vi "Configure Measurement Trend (TIE).vi"(0 "VISA resource name":refnum<visa-resource-name>, 1 "Enable Measurement Trend (T:Enable)":bool, 2 "Direction (0: Rising)":i32(ring) items=["Rising", "Falling", "Both"], 3 "Units (0: Second)":i32(ring) items=["Second", "Unit Interval"], 5 "Source 1 (1: Channel 1)":i32(ring) items=["Channel 1", "Channel 2", "Channel 3", "Channel 4", "Function 1", "Function 2", "Function 3", "Function 4", "Memory 1", "Memory 2", "Memory 3", "Memory 4"], 9 "Measurement Function (0: Time Interval Error (Data))":i32(ring) items=["Time Interval Error (Data)", "Time Interval Error (Clock)"], 11 "error in (no error)":errorcluster) -> (4 "VISA resource name out":refnum<visa-resource-name>, 15 "error out":errorcluster)   [LabVIEW 2009, in "Agilent 8000 Series.lvlib"]
doc: "Configures either Time Interval Error measurement and enables the Measurement Trend Jitter analysis on it.\n\n<B>Note:</B>\nCalling this VI disables all previously enabled measurements and clears existing measurement results from display."
uses:
  Agilent 8000 Series.lvlib
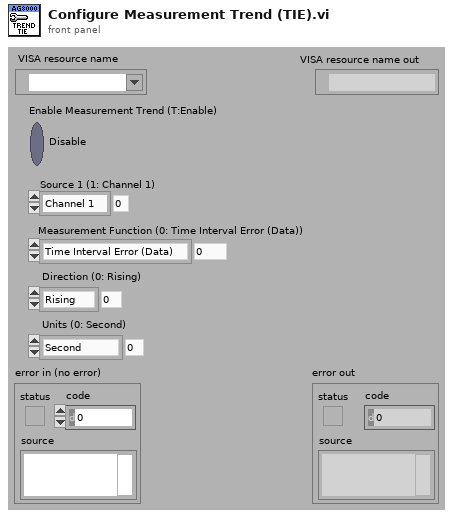
[diagram p1: front panel]
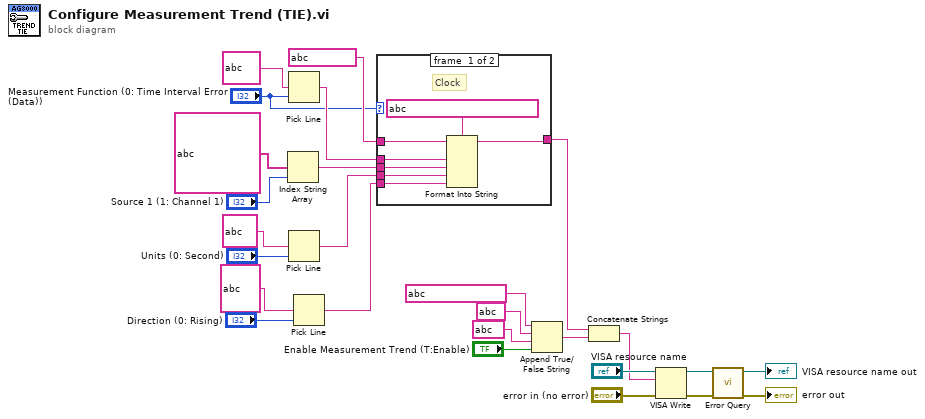
[diagram p0: block diagram]
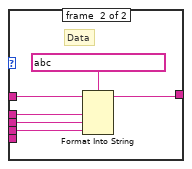
[diagram p2: hidden frame]
diagram:
  n1 = Index String Array(1:"Source 1 (1: Channel 1)", 2:string[] ?) -> (0:w15:string)  [unwired: 1 in]
  n2 = Pick Line(multi-line string=string ?, line index="Measurement Function (0: Time Interval Error (Data))") -> (output string=w18:string)  [unwired: 1 in]
  n3 = Pick Line(multi-line string=string ?, line index="Units (0: Second)") -> (output string=w9:string)  [unwired: 1 in]
  n4 = Pick Line(multi-line string=string ?, line index="Direction (0: Rising)") -> (output string=w8:string)  [unwired: 1 in]
  n5 = case shown="0, Default" "Measurement Function (0: Time Interval Error (Data))" {
    tunnel: string ? ("initial string") -> [w33 w39]
    tunnel: w18 -> [w31 w37]
    tunnel: w15 -> [w30 w36]
    tunnel: [w29 w35] -> w2
    tunnel: w9 -> [w28 w34]
    tunnel: w8 -> [w27 _]
    frame #0 {
      # "Clock"
      n6 = Format Into String(format string=string ?, initial string=w33, w31, w30, w28, w27) -> (resulting string=w29:string)  [unwired: 1 in, 1 out]
    }
    frame #1 {
      # "Data"
      n7 = Format Into String(format string=string ?, initial string=w39, w37, w36, w34) -> (resulting string=w35:string)  [unwired: 1 in, 1 out]
    }
  }
  n8 = Append True/False String(1:"Enable Measurement Trend (T:Enable)", 2:string ? ("false string"), 3:string ? ("true string"), 4:string ? ("string (\"\")")) -> (0:w3:string)
  n9 = Concatenate Strings(w2, w3) -> (w1:string)
  n10 = VISA Write(VISA resource name="VISA resource name", write buffer=w1, error in (no error)="error in (no error)") -> (VISA resource name out=w22:refnum<visa-resource-name>, error out=w21:errorcluster)  [unwired: 1 out]
  n11 = call "Error Query.vi"("error in (no error)"=w21, "VISA resource name"=w22) -> ("error out"=→"error out":errorcluster, "VISA resource name out"=→"VISA resource name out":refnum<visa-resource-name>)  [unwired: 6 in, 2 out]
